vi "count.vi"(6 "quein?":bool=TRUE, 8 "error in (no error)":errorcluster, 11 "py in":T1) -> (0 "error out":errorcluster, 2 "count":i32, 3 "py out":T1)   [LabVIEW 2022 SP3, in "pythonq.lvlib"]
uses:
  pythonq.lvlib
  py_session.ctl
  py_cluster.ctl
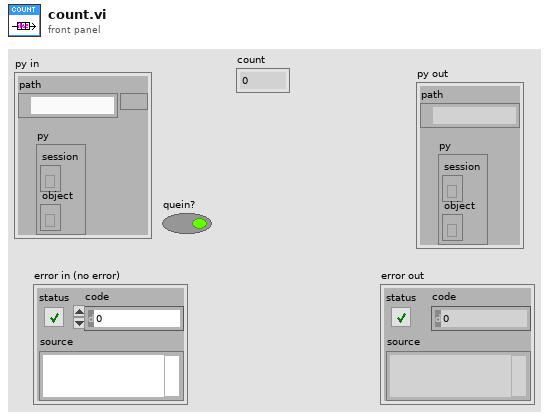
[diagram p1: front panel]
types:
  T1 = typedef "pythonq.lvlib/py_cluster.ctl" = cluster{"path":path, "py":T2}
  T2 = typedef "pythonq.lvlib/py_session.ctl" = cluster{"session":refnum<k35>, "object":refnum<k38>}
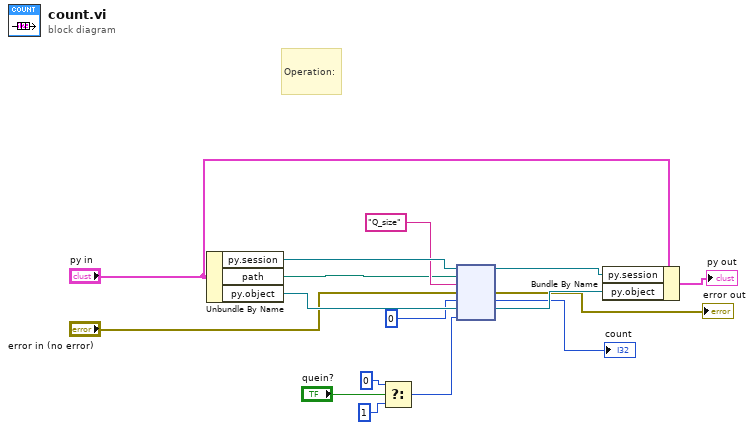
[diagram p0: block diagram]
diagram:
  # "Operation:"
  n1 = Unbundle By Name("py in") -> ("py.session"=w15:refnum<k35>, "path"=w9:path, "py.object"=w16:refnum<k38>)
  n2 = Select(t=0, s="quein?", f=1) -> (s? t:f=w2:i32)
  n3 = node(w15, w9, "Q_size" ("function name"), "error in (no error)", 0, w16, w2) -> (w12:refnum<k35>, →"error out":errorcluster, →"count":i32, w11:refnum<k38>)  [unwired: 1 in, 2 out]
  n4 = Bundle By Name(cluster="py in", "py.session"=w12, "py.object"=w11) -> (→"py out":T1)
